vi "1.vi"() -> ()   [LabVIEW 2017]
panel:
  out "y":dbl=20.0 format="%#_13g"
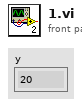
[diagram p1: front panel]
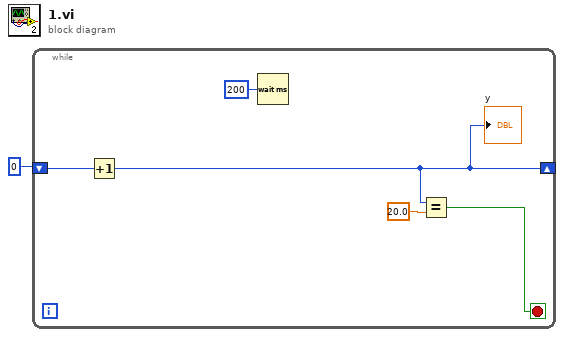
[diagram p0: block diagram]
diagram:
  n1 = while {
    shift-right: [w2] -> _
    shift-left: u32 0 ("milliseconds to wait") -> [w6]
    stop <- w3 stop-if-true
    n2 = Increment(x=w6) -> (x+1=w2:u32)
    "y" <- w2
    n3 = Wait (ms)(milliseconds to wait=u32 200) -> ()  [unwired: 1 out]
    n4 = Equal?(x=w2, y=20.0) -> (x = y?=w3:bool)
  }
